vi "Periodic Tasks.vi"() -> ()   [LabVIEW 2012]
doc: "This VI runs in parallel to other tasks. It can contain as many user-defined periodic loops as you need. These can carry out PID or other sorts of timed response."
uses:
  <vilib>/Rock Robotics/SystemInterfaces/Utilities/FPGA_UtilitiesLED Source.ctl
  <vilib>/Rock Robotics/SystemInterfaces/Utilities/FPGA_UtilitiesLED State.ctl
  Robot Global Data.vi
panel:
  out "Heading":dbl
  out "Rate":dbl
  out "Distance":dbl
  out "Angular Rate":dbl
  out "Angle":dbl
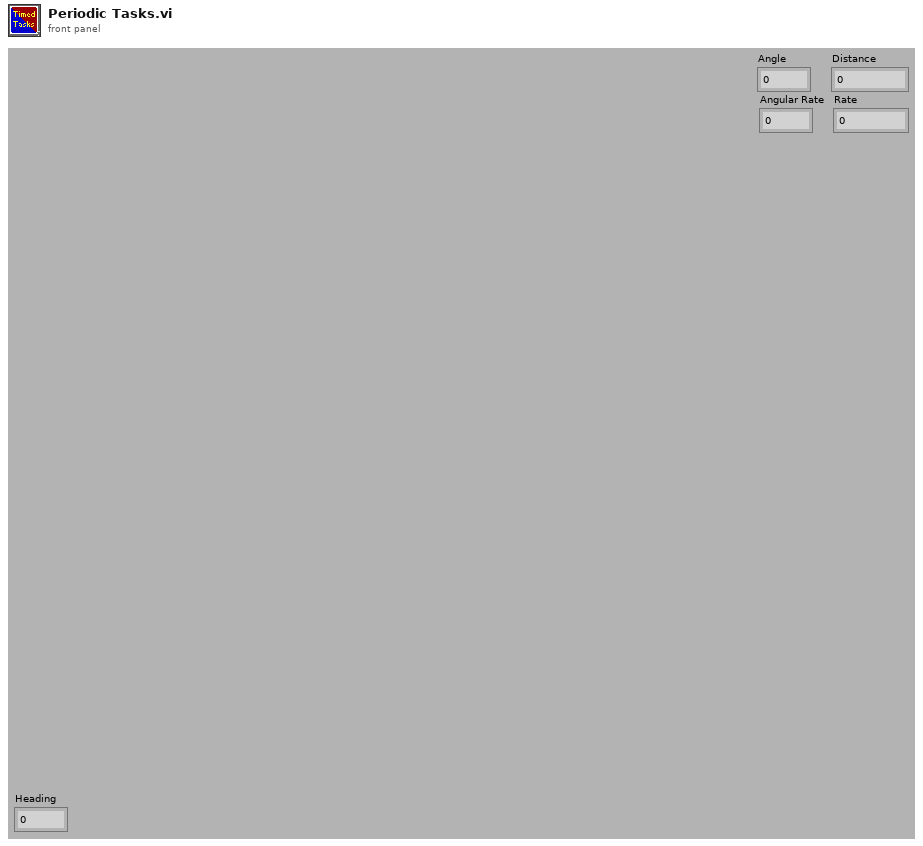
[diagram p1: front panel]
types:
  T1 = typedef "FPGA_UtilitiesLED State.ctl" = enum16{"Off", "On", "Toggle"}
  T2 = typedef "FPGA_UtilitiesLED Source.ctl" = enum16{"User LED", "FPGA LED"}
  T3 = typedef "WPI_I2CDevRef.ctl" = cluster{"DevStatus":errorcluster, "Digital Module":T4, "Device Address":u8}
  T4 = typedef "FPGA_TypedefDigitalModule.ctl" = enum16{"Digital Module 1", "Digital Module 2"}
  T5 = typedef "WPI_GyroDevRef.ctl" = cluster{"DevStatus":errorcluster, "Analog Module":T6, "Analog Channel":T7, "Offset":dbl, "Gain (VoltsPerDegree/Second)":dbl}
  T6 = typedef "FPGA_TypedefAnalogModule.ctl" = enum16{"Analog Module 1", "Analog Module 2"}
  T7 = typedef "FPGA_AIChannel.ctl" = enum8{"AI 1", "AI 2", "AI 3", "AI 4", "AI 5", "AI 6", "AI 7", "AI 8", "Invalid"}
  T8 = typedef "WPI_EncoderDevRef.ctl" = cluster{"DevStatus":errorcluster, "EncoderIndex":T9, "CounterIndex":T10, "DistancePerCount":dbl, "Decoding Type":T11}
  T9 = typedef "FPGA_EncoderIdx.ctl" = enum8{"Enc 0", "Enc 1", "Enc 2", "Enc 3", "Invalid"}
  T10 = typedef "FPGA_CounterCtrSystemIndex.ctl" = enum8{"Ctr 0", "Ctr 1", "Ctr 2", "Ctr 3", "Ctr 4", "Ctr 5", "Ctr 6", "Ctr 7", "Invalid"}
  T11 = typedef "WPI_EncoderType.ctl" = enum16{"1x", "2x", "4x"}
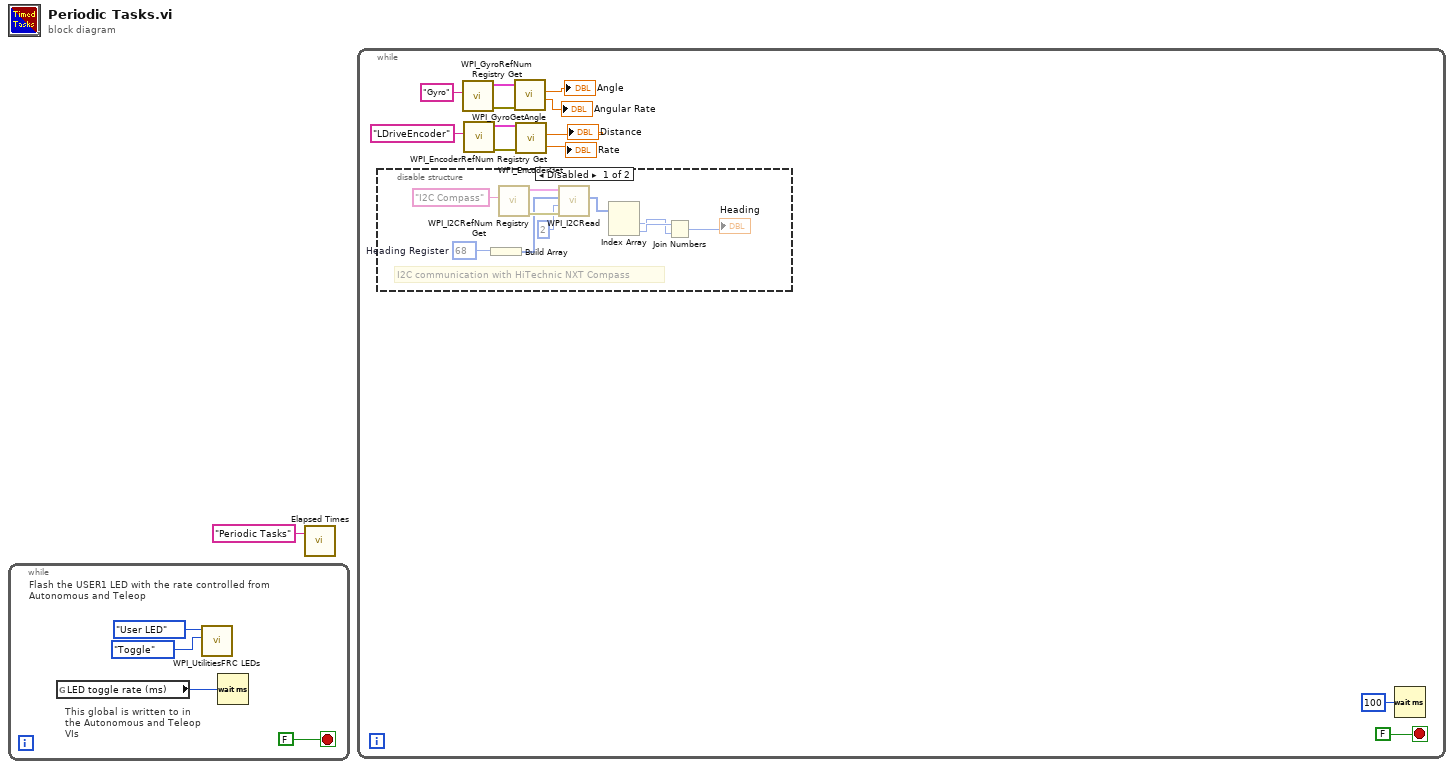
[diagram p0: block diagram]
diagram:
  n1 = while {
    stop <- FALSE stop-if-true
    # "This global is written to in the Autonomous and Teleop VIs"
    # "Flash the USER1 LED with the rate controlled from Autonomous and Teleop"
    n2 = global read "Robot Global Data.vi" "LED toggle rate (ms)"() -> (w2:u32)
    n3 = call <vilib>:"WPI_UtilitiesFRC LEDs.vi"("State"=FPGA_UtilitiesLED_State."Toggle", "LED Type"=FPGA_UtilitiesLED_Source."User LED") -> ()  [unwired: 1 in, 9 out]
    n4 = Wait (ms)(milliseconds to wait=w2) -> ()  [unwired: 1 out]
  }
  n5 = call "Elapsed Times.vi"("Call Name"="Periodic Tasks") -> ()  [unwired: 2 in, 1 out]
  n6 = while {
    stop <- FALSE stop-if-true
    n7 = disable-structure shown="Disabled" {
      frame Disabled {
        w24 = u8 68  # Heading Register
        # "I2C communication with HiTechnic NXT Compass"
        n8 = Build Array(w24) -> (w23:u8[])
        n9 = call <vilib>:"WPI_I2CRefNum Registry Get.vi"("refnum name"="I2C Compass") -> ("error out"=w26:errorcluster, "I2CDevRef"=w25:T3)  [unwired: 9 in]
        n10 = call <vilib>:"WPI_I2CRead.vi"("error in (no error)"=w26, "I2CBytesToRead"=u8 2, "I2CRegister"=w23, "I2CDevRef"=w25) -> ("Data Out"=w21:u8[])  [unwired: 5 in, 2 out]
        n11 = Index Array(array=w21) -> (element #1=w19:u8, element #2=w20:u8)  [unwired: 2 in]
        n12 = Join Numbers(hi=w20, lo=w19) -> ((hi.lo)=→"Heading":u16)
      }
      frame Enabled {
      }
    }
    n13 = call <vilib>:"WPI_GyroRefNum Registry Get.vi"("refnum name"="Gyro") -> ("error out"=w8:errorcluster, "GyroDevRef"=w9:T5)  [unwired: 9 in]
    n14 = call <vilib>:"WPI_EncoderRefNum Registry Get.vi"("refnum name"="LDriveEncoder") -> ("error out"=w6:errorcluster, "EncoderDevRef"=w7:T8)  [unwired: 9 in]
    n15 = call <vilib>:"WPI_GyroGetAngle.vi"("error in (no error)"=w8, "GyroDevRef"=w9) -> ("Angular Rate"=→"Angular Rate":dbl, "Angle"=→"Angle":dbl)  [unwired: 6 in, 2 out]
    n16 = call <vilib>:"WPI_EncoderGet.vi"("error in (no error)"=w6, "EncoderDevRef"=w7) -> ("Distance"=→"Distance":dbl, "Rate"=→"Rate":dbl)  [unwired: 4 in, 4 out]
    n17 = Wait (ms)(milliseconds to wait=u32 100) -> ()  [unwired: 1 out]
  }
